vi "Do Callback.vi"(8 "error in (no error)":errorcluster, 10 "Numeric":dbl, 11 "Callback Producer in":refnum<class "Callback Producer.lvclass">) -> (0 "error out":errorcluster, 3 "Callback Producer out":refnum<class "Callback Producer.lvclass">)   [LabVIEW 2020, in "Callback Producer.lvclass"]
uses:
  Callback Producer.lvclass
  Callback Producer.lvclass/Callback Producer.ctl
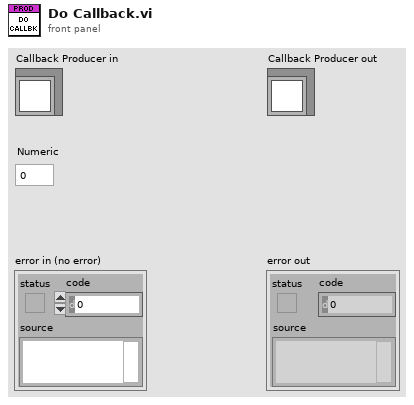
[diagram p1: front panel]
types:
  T1 = typedef "Callback Producer.lvclass/Ref Data.ctl" = cluster{"Callbacks":T2[]}
  T2 = typedef "Callback Producer.lvclass/Callback.ctl" = cluster{"Owner":refnum<class>, "VI":refnum<vi>}
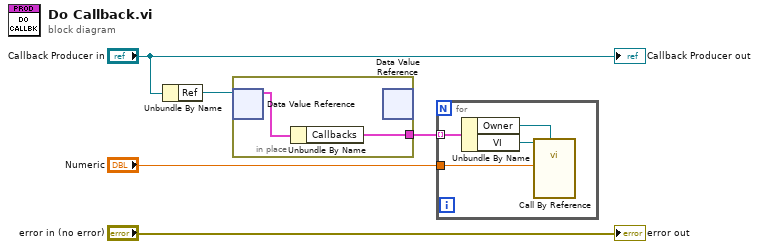
[diagram p0: block diagram]
diagram:
  n1 = Unbundle By Name("Callback Producer in") -> ("Ref"=w4:refnum<data-value>)
  n2 = in-place {
    in-place-border: [w6] -> w2
    n3 = in-place-dvr #1(w4) -> (w7:T1)  [unwired: 1 out]
    n4 = Unbundle By Name(w7) -> ("Callbacks"=w6:T2[])
    n5 = in-place-dvr #1() -> ()  [unwired: 1 in, 2 out]
  }
  n6 = for {
    tunnel: w2 -> [w11] mode=indexing
    tunnel: "Numeric" -> [w8]
    n7 = Unbundle By Name(w11) -> ("Owner"=w9:refnum<class>, "VI"=w10:refnum<vi>)
    n8 = call-by-ref "?"(reference=w10, "Owner"=w9, "Numeric"=w8) -> ()  [unwired: 11 in, 2 out]
  }
  "error out" <- "error in (no error)"
  "Callback Producer out" <- "Callback Producer in"
